vi "configure assembly.vi"(8 "error in":errorcluster, 10 "assembly definition in":T2={"name"="", "Instance ID"=100, "Type"=enum."Producing", "Size (bytes)"=32}, 11 "EthernetIP configuration":refnum<class "EthernetIP configuration.lvclass">) -> (0 "error out":errorcluster, 1 "success":bool, 2 "assembly definition out":T2={"name"="", "Instance ID"=100, "Type"=enum."Producing", "Size (bytes)"=32}, 5 "changed":bool)   [LabVIEW 2013, in "EthernetIP editor node.lvclass"]
uses:
  EthernetIP editor node.lvclass
  <vilib>/NI/TBM Modules/Ethernet IP/configuration/EthernetIP configuration.lvclass
  <vilib>/NI/TBM Modules/Ethernet IP/configuration/assembly definition.ctl
  <vilib>/NI/TBM Modules/Ethernet IP/configuration/assembly type.ctl
  <vilib>/NI/TBM Modules/Ethernet IP/configuration/EthernetIP configuration.lvclass/EthernetIP configuration.ctl
  <vilib>/NI/TBM Modules/Ethernet IP/configuration/Read assemblies.vi
panel:
  in  "Size (bytes)":u32
  in  "Instance ID":u32
  in  "Asm Type":T1
  in  "Assembly Name (opt)":string
  in  "cancel":bool
  in  "ok":bool
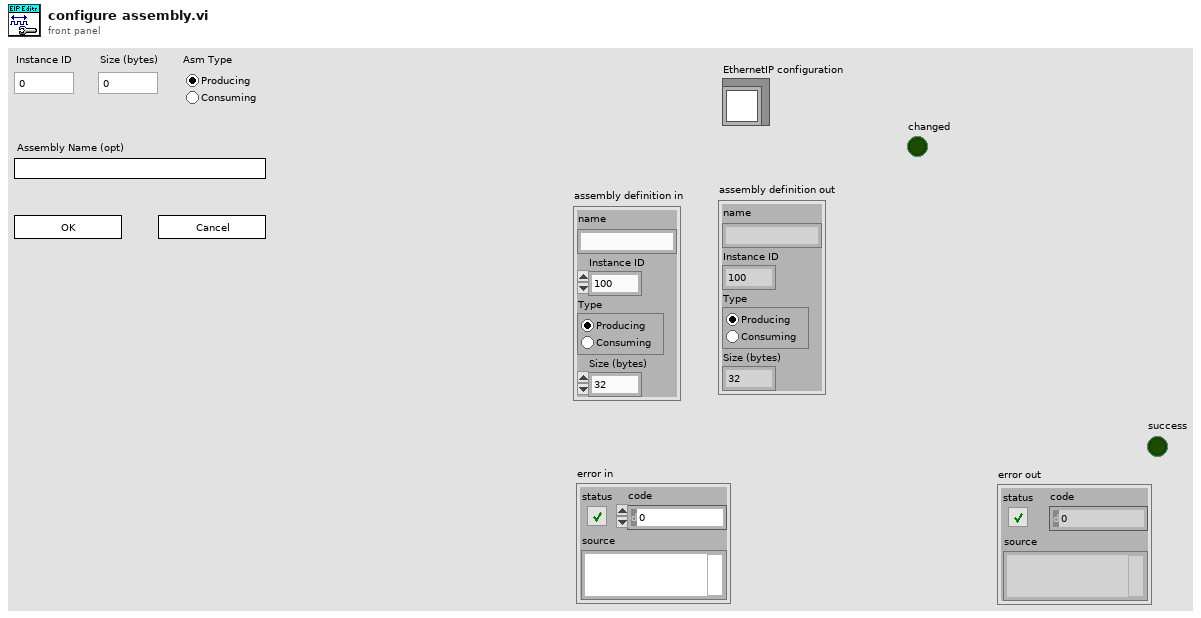
[diagram p1: front panel]
types:
  T1 = typedef "EthernetIP configuration.lvclass/assembly type.ctl" = enum32{"Producing", "Consuming"}
  T2 = typedef "EthernetIP configuration.lvclass/assembly definition.ctl" = cluster{"name":string, "Instance ID":u32, "Type":T1, "Size (bytes)":u32}
  T3 = enum32{"Invalid", "Standard", "Closed", "Hidden", "Minimized", "Maximized"}
  T4 = enum32{"Invalid", "Default", "Floating", "Floating/Auto-Hide", "Modal"}
  T5 = enum32{"invalid app kind", "Development System", "Run Time System", "Student Edition", "Embedded LabVIEW", "Evaluation", "Custom"}
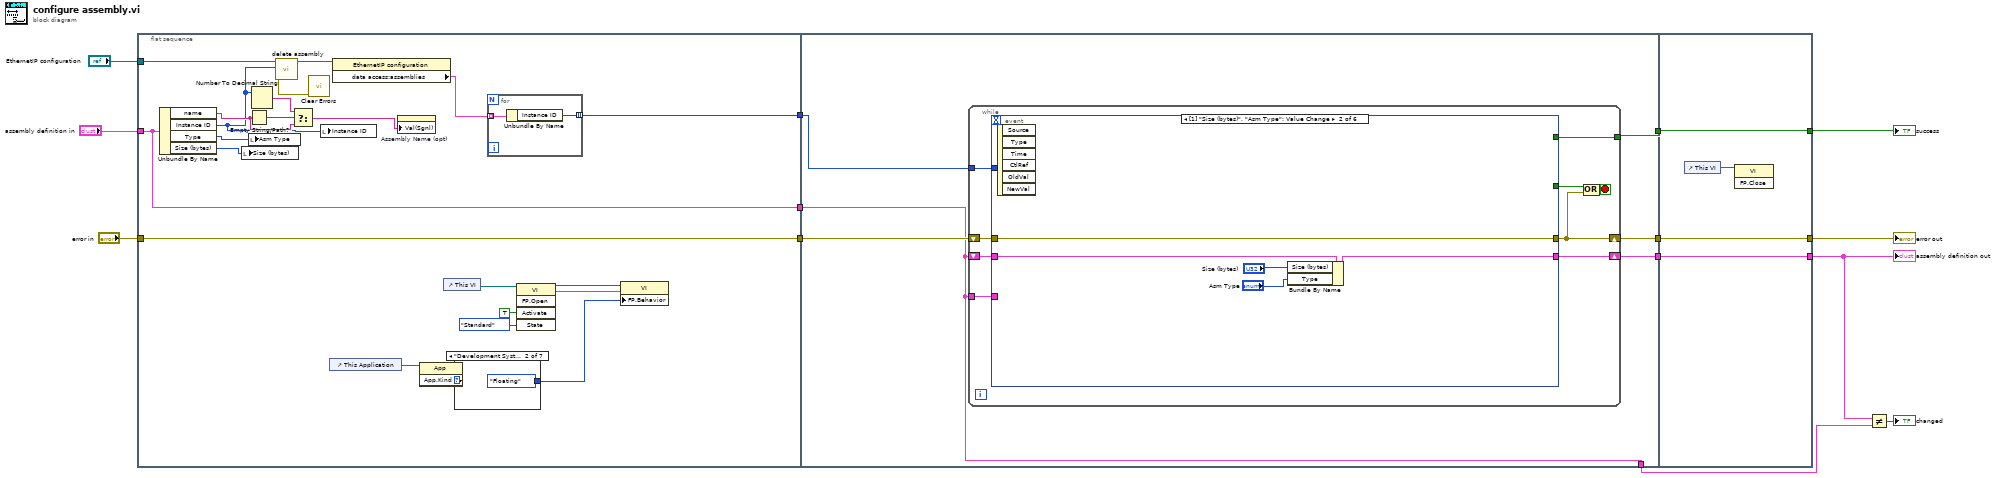
[diagram p0: block diagram]
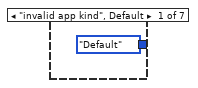
[diagram p2: hidden frame]
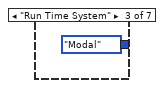
[diagram p3: hidden frame]
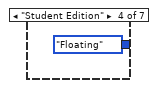
[diagram p4: hidden frame]
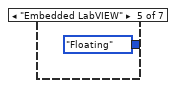
[diagram p5: hidden frame]
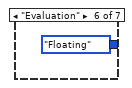
[diagram p6: hidden frame]
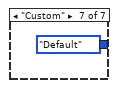
[diagram p7: hidden frame]
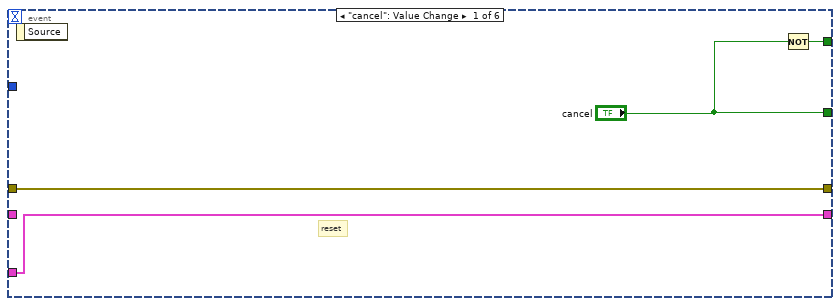
[diagram p8: hidden frame]
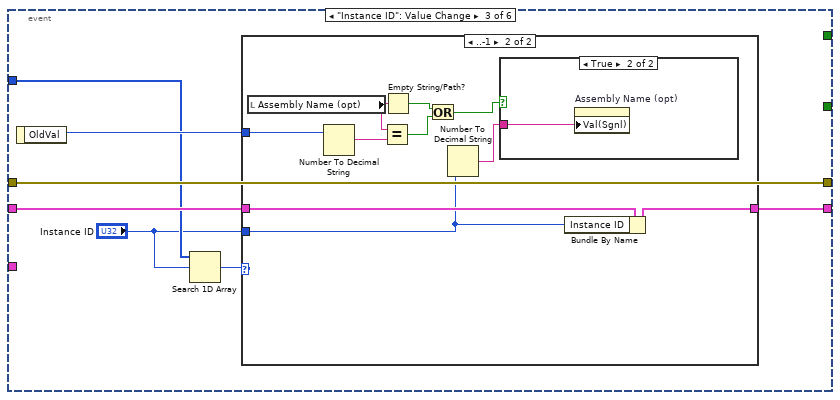
[diagram p9: hidden frame]
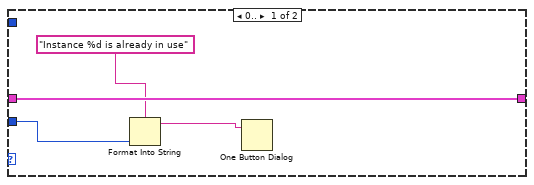
[diagram p10: hidden frame]
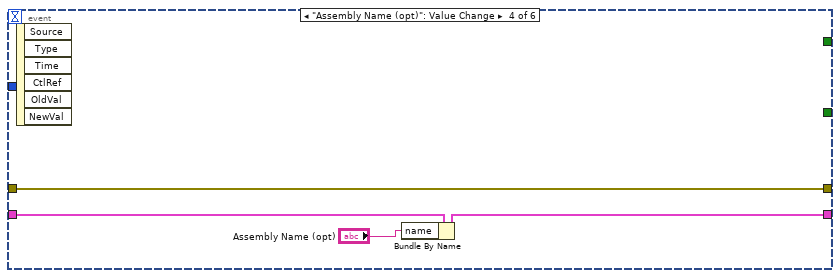
[diagram p12: hidden frame]
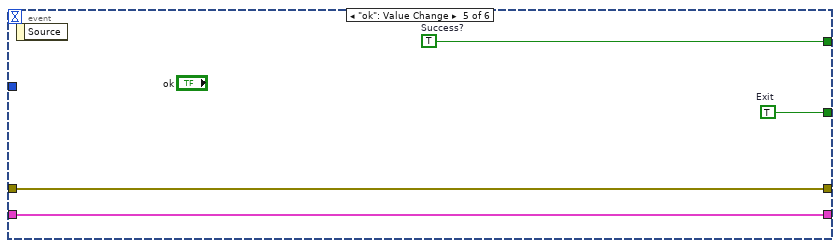
[diagram p13: hidden frame]
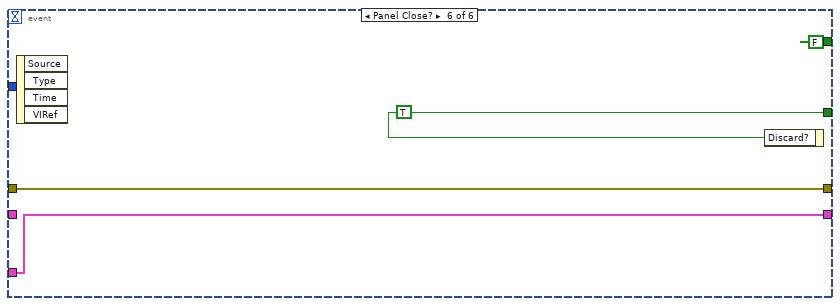
[diagram p14: hidden frame]
diagram:
  n1 = flat-sequence {
    tunnel: "error in" -> [w20]
    tunnel: "EthernetIP configuration" -> [w28]
    tunnel: "assembly definition in" -> [w16]
    tunnel: [w24] -> w5
    tunnel: [w20] -> w4
    tunnel: [w16] -> w3
    tunnel: [w51] -> w10
    tunnel: [w50] -> w9
    tunnel: [w49] -> w8
    tunnel: w5 -> [w46]
    tunnel: w4 -> [w48]
    tunnel: w3 -> [w47]
    tunnel: [w47] -> w2
    tunnel: [w105] -> w1
    tunnel: [w106] -> w12
    tunnel: [w107] -> w13
    tunnel: w10 -> [w107]
    tunnel: w9 -> [w106]
    tunnel: w8 -> [w105]
    frame #0 {
      n2 = Unbundle By Name(w16) -> ("name"=w22:string, "Instance ID"=w18:u32, "Type"=w19:T1, "Size (bytes)"=w17:u32)
      n3 = local write "Size (bytes)"(w17) -> ()
      n4 = local write "Asm Type"(w19) -> ()
      n5 = Empty String/Path?(string/path=w22) -> (empty?=w23:bool)
      n6 = Number To Decimal String(number=w18) -> (decimal integer string=w21:string)  [unwired: 1 in]
      n7 = call <vilib>:"delete assembly.vi"("instance ID"=w18, "EthernetIP configuration in"=w28) -> ("error out"=w25:errorcluster, "EthernetIP configuration out"=w26:refnum<class "EthernetIP configuration.lvclass">)  [unwired: 7 in, 1 out]
      n8 = Select(t=w21, s=w23, f=w22) -> (s? t:f=w15:string)
      n9 = call <vilib>:"Clear Errors.vi"("error in (no error)"=w25) -> ()  [unwired: 6 in, 1 out]
      n10 = local write "Instance ID"(w18) -> ()
      n11 = control-ref of="This Application"() -> (w31:refnum<vi>)
      n12 = property class="EthernetIP configuration"(reference=w26) -> ("data access:assemblies"=w27:T2[])  [unwired: 1 in, 2 out]
      n13 = property on="Assembly Name (opt)" class="Str"("Val(Sgnl)"=w15) -> ()  [unwired: 2 in, 2 out]
      n14 = property class="App"(reference=w31) -> ("App.Kind"=w30:T5)  [unwired: 1 in, 2 out]
      n15 = control-ref of="This VI"() -> (w32:refnum<vi>)
      n16 = case shown="\"Development System\"" w30 {
        tunnel: [T4."Default" ("Front Panel Window:Behavior") T4."Floating" ("Front Panel Window:Behavior") T4."Modal" ("Front Panel Window:Behavior") T4."Floating" ("Front Panel Window:Behavior") T4."Floating" ("Front Panel Window:Behavior") T4."Floating" ("Front Panel Window:Behavior") T4."Default" ("Front Panel Window:Behavior")] -> w29
        frame "invalid app kind", Default {
        }
        frame "Development System" {
        }
        frame "Run Time System" {
        }
        frame "Student Edition" {
        }
        frame "Embedded LabVIEW" {
        }
        frame "Evaluation" {
        }
        frame "Custom" {
        }
      }
      n17 = for {
        tunnel: w27 -> [w38] mode=indexing
        tunnel: [w37] -> w24 mode=indexing
        n18 = Unbundle By Name(w38) -> ("Instance ID"=w37:u32)
      }
      n19 = invoke class="VI" method="FP.Open"(reference=w32, "Activate"=TRUE ("Activate?"), "State"=T3."Standard") -> (reference out=w35:refnum<vi>, error out=w36:errorcluster)  [unwired: 2 in, 3 out]
      n20 = property class="VI"(reference=w35, error in=w36, "FP.Behavior"=w29) -> ()  [unwired: 2 out]
    }
    frame #1 {
      n21 = while {
        shift-right: [w55] -> w50
        shift-left: w48 -> [w60]
        tunnel: [w59] -> w51
        shift-right: [w53] -> w49
        shift-left: w47 -> [w56]
        tunnel: w47 -> [w54]
        tunnel: w46 -> [w52]
        stop <- w57 stop-if-true
        n22 = event shown="[1] \"Size (bytes)\", \"Asm Type\": Value Change" {
          selector: _ -> [_ _ _ _ _ _]
          dyn-events: _ -> [_ _ _ _ _ _]
          timeout: _ -> [_ _ _ _ _ _]
          tunnel: w60 -> [w64 w69 w76 w95 w99 w103]
          tunnel: [w64 w69 w76 w95 w99 w103] -> w55
          tunnel: [w63 _ _ _ w96 FALSE] -> w59
          tunnel: ["cancel" _ _ _ w97 w101] -> w58
          tunnel: w56 -> [_ w68 w75 w94 w98 _]
          tunnel: [w61 w67 w74 w93 w98 w100] -> w53
          tunnel: w54 -> [w61 _ _ _ _ w100]
          tunnel: w52 -> [_ _ w72 _ _ _]
          event "cancel": Value Change {
            # "reset"
            n23 = event-data() -> ()  [unwired: 1 in, 1 out]
            n24 = Not(x="cancel") -> (.not. x?=w63:bool)
          }
          event "Size (bytes)": Value Change {
            n25 = event-data() -> ()  [unwired: 1 in, 6 out]
            n26 = Bundle By Name(cluster=w68, "Size (bytes)"="Size (bytes)", "Type"="Asm Type") -> (w67:T2)
          }
          event "Instance ID": Value Change {
            n27 = event-data() -> ("OldVal"=w73:u32)  [unwired: 1 in]
            n28 = Search 1D Array(1D array=w72, element="Instance ID") -> (index of element=w70:i32)  [unwired: 1 in]
            n29 = case shown="..-1" w70 {
              tunnel: w75 -> [w80 w90]
              tunnel: [w80 w89] -> w74
              tunnel: w73 -> [_ w88]
              tunnel: "Instance ID" -> [w79 w81]
              frame 0.. {
                n30 = Format Into String(format string="Instance %d is already in use", w79) -> (resulting string=w78:string)  [unwired: 2 in, 1 out]
                n31 = One Button Dialog(message=w78) -> ()  [unwired: 1 in, 1 out]
              }
              frame ..-1 {
                n32 = local read "Assembly Name (opt)"() -> (w84:string)
                n33 = Number To Decimal String(number=w88) -> (decimal integer string=w85:string)  [unwired: 1 in]
                n34 = Equal?(x=w84, y=w85) -> (x = y?=w86:bool)
                n35 = Empty String/Path?(string/path=w84) -> (empty?=w87:bool)
                n36 = Or(x=w87, y=w86) -> (x .or. y?=w83:bool)
                n37 = Number To Decimal String(number=w81) -> (decimal integer string=w82:string)  [unwired: 1 in]
                n38 = case shown="True" w83 {
                  tunnel: w82 -> [_ w91]
                  frame False {
                  }
                  frame True {
                    n39 = property on="Assembly Name (opt)" class="Str"("Val(Sgnl)"=w91) -> ()  [unwired: 2 in, 2 out]
                  }
                }
                n40 = Bundle By Name(cluster=w90, "Instance ID"=w81) -> (w89:T2)
              }
            }
          }
          event "Assembly Name (opt)": Value Change {
            n41 = event-data() -> ()  [unwired: 1 in, 6 out]
            n42 = Bundle By Name(cluster=w94, "name"="Assembly Name (opt)") -> (w93:T2)
          }
          event "ok": Value Change {
            w96 = TRUE  # Success?
            w97 = TRUE  # Exit
            n43 = event-data() -> ()  [unwired: 1 in, 1 out]
          }
          event Panel Close? {
            w101 = TRUE ("cancel")
            n44 = event-data() -> ()  [unwired: 1 in, 4 out]
            n45 = event-data("Discard?"=w101) -> ()  [unwired: 1 in, 1 out]
          }
        }
        n46 = Compound Arithmetic op=OR(w58, w55) -> (w57:bool)
      }
    }
    frame #2 {
      n47 = control-ref of="This VI"() -> (w104:refnum<vi>)
      n48 = invoke class="VI" method="FP.Close"(reference=w104) -> ()  [unwired: 2 in, 3 out]
    }
  }
  n49 = Not Equal?(x=w1, y=w2) -> (x != y?=→"changed":bool)
  "error out" <- w12
  "success" <- w13
  "assembly definition out" <- w1
